vi "Server_CleanUp.vi"(8 "error in (no error)":errorcluster) -> (0 "error out":errorcluster)   [LabVIEW 2023, in "Server.lvclass"]
uses:
  Server.lvclass
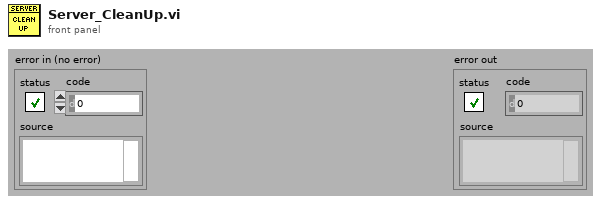
[diagram p1: front panel]
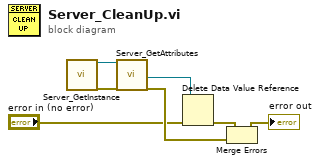
[diagram p0: block diagram]
diagram:
  n1 = call "Server_GetInstance.vi"() -> ("reference out"=w5:refnum<class "Server.lvclass">, "error out"=w6:errorcluster)  [unwired: 15 in, 3 out]
  n2 = call "Server_GetAttributes.vi"("reference in"=w5, "error in (no error)"=w6) -> ("DataRef"=w2:refnum<data-value>, "error out"=w4:errorcluster)  [unwired: 14 in, 2 out]
  n3 = Delete Data Value Reference(data value reference=w2, error in="error in (no error)") -> (error out=w1:errorcluster)  [unwired: 1 out]
  n4 = Merge Errors(w1, w4) -> (→"error out":errorcluster)
